vi "Write measurement.hardware[].timestamp.vi"(8 "error in (no error)":errorcluster, 10 "measurement.hardware[].timestamp":string, 11 "Results in":refnum<class "Results.lvclass">) -> (0 "error out":errorcluster, 3 "Results out":refnum<class "Results.lvclass">)   [LabVIEW 2015, in "Result Actor.lvlib" / "Results.lvclass"]
uses:
  Results.lvclass
  Results.lvclass/Results.ctl
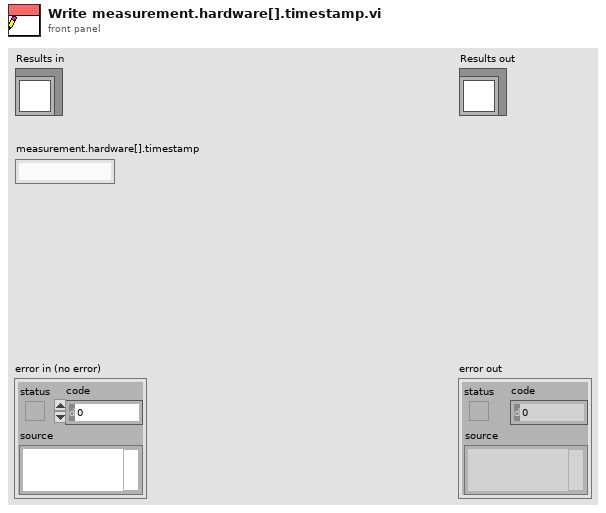
[diagram p1: front panel]
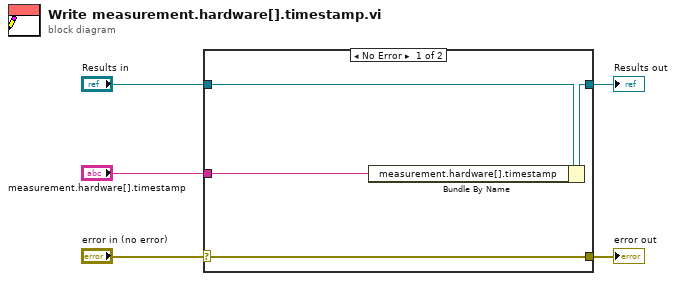
[diagram p0: block diagram]
diagram:
  n1 = case shown="No Error" "error in (no error)" {
    selector: "error in (no error)" -> [w9 w10]
    tunnel: [w9 w10] -> w4
    tunnel: [w7 w11] -> w2
    tunnel: "Results in" -> [w8 w11]
    tunnel: "measurement.hardware[].timestamp" -> [w6 _]
    frame No Error {
      n2 = Bundle By Name(cluster=w8, "measurement.hardware[].timestamp"=w6) -> (w7:refnum<class "Results.lvclass">)
    }
    frame Error {
    }
  }
  "error out" <- w4
  "Results out" <- w2
